vi "Test_API_AsynchShutdown_NoErrorEventsCaptured.vi"(8 "error in (no error)":errorcluster, 11 "TestCase in":refnum<class "TestLocalLogInstance.lvclass">) -> (0 "error out":errorcluster, 3 "TestCase out":refnum<class "TestLocalLogInstance.lvclass">)   [LabVIEW 2019, in "TestLocalLogInstance.lvclass"]
uses:
  TestLocalLogInstance.lvclass
  Source/Composed Log/Types/Log Level.ctl
  Source/LVQueue Sink/LVQueue Sink.lvclass/LVQueue Sink.ctl
  Source/Composed Log/LoggerReference/LoggerReference.lvclass/LoggerReference.ctl
  e881e85d-d289-450a-a3bf-8e76de4143bc.vi
  145e8f28-aa7d-4165-8971-95667389dd01.vi
  Source/Composed Log/LoggerReference/Return Aggregate Queues.vi
  Source/Composed Log/LoggerReference/Add Aggregate Log.vi
  e881e85d-d289-450a-a3bf-8e76de4143bc.vi/56849bd9-e0f3-42e2-9e62-1194216846a3.vi
  Source/Composed Log/LoggerReference/Log.vi
  Source/Composed Log/LoggerReference/Get Valid Event Time.vi
  Source/Composed Log/LoggerReference/Send Add Sink.vi
  Source/Composed Log/LoggerReference/Remove Stale Logs.vi
  Source/LVQueue Sink/LVQueue Sink.lvclass
  C:/CS/Log/Source/Composed Log/Log Sink/Log Sink.lvclass
  Source/Composed Log/Application Logger/Launch Worker Loop.vi
  Source/Composed Log/LoggerReference/Initialize Logger Instance.vi
  Source/Composed Log/LoggerReference/LoggerReference.lvclass
  Source/Composed Log/IErrorFormat/IErrorFormat.lvclass
  Source/Composed Log/Log Sink/Log Sink.lvclass
  <vilib>/addons/_JKI Toolkits/VI Tester/TestCase.llb/TestCase.lvclass
  Source/Composed Log/Composed Log.lvlib
  C:/Program Files (x86)/National Instruments/LabVIEW 2019/vi.lib/addons/_JKI Toolkits/VI Tester/TestCase.llb/TestCase.lvclass
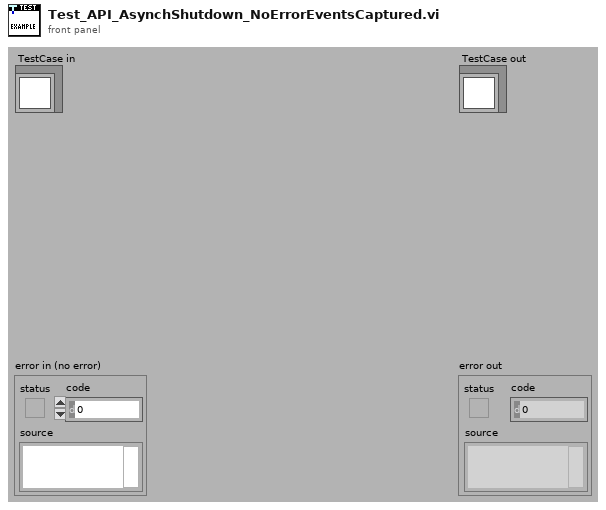
[diagram p1: front panel]
types:
  T1 = typedef "Composed Log.lvlib/Log Level.ctl" = enum16{"Debug", "Info", "Warning", "Error", "Critical"}
  T2 = typedef "Composed Log.lvlib/Log Packet.ctl" = cluster{"Data To Log":string, "Source":string, "Event Level":T1, "Event Time":timestamp}
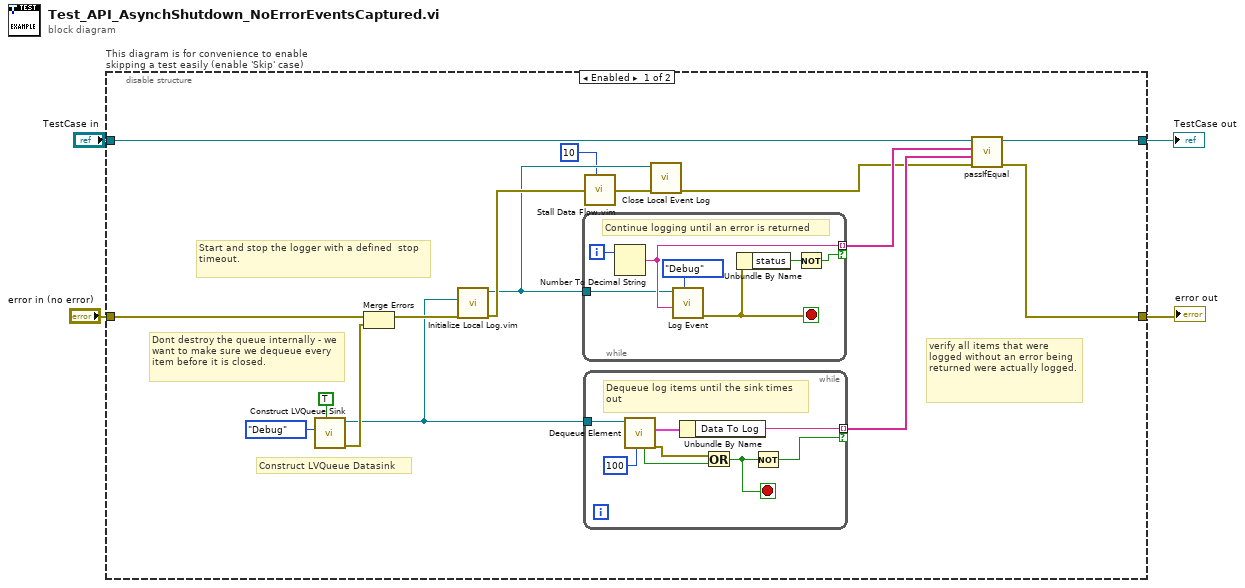
[diagram p0: block diagram]
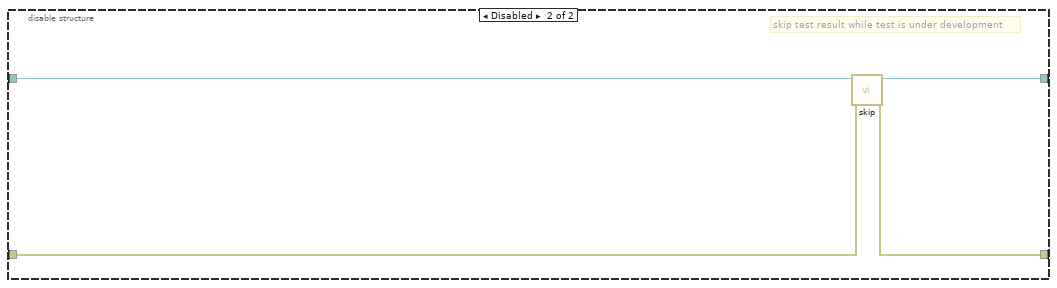
[diagram p2: hidden frame]
diagram:
  n1 = disable-structure "This diagram is for convenience to enable skipping a test easily (enable 'Skip' case)" shown="Enabled" {
    disable-tunnel: "TestCase in" -> [w18 w39]
    disable-tunnel: [w19 w37] -> w1
    disable-tunnel: [w17 w38] -> w3
    disable-tunnel: "error in (no error)" -> [w20 w36]
    frame Enabled {
      # "Dont destroy the queue internally - we want to make sure we dequeue every item before it is closed."
      # "verify all items that were logged without an error being returned were actually logged."
      # "Construct LVQueue Datasink"
      # "Start and stop the logger with a defined  stop timeout."
      n2 = call "Construct LVQueue Sink.vi"("User Shutdown? (F)"=TRUE, "LogLevel"=Log_Level."Debug") -> ("error out"=w15:errorcluster, "LVQueue Sink out"=w10:refnum<class "LVQueue Sink.lvclass">)  [unwired: 8 in]
      n3 = Merge Errors(w20, w15) -> (w11:errorcluster)
      n4 = call "Initialize Local Log.vim"("error in (no error)"=w11, "Startup Sink(s)"=w10) -> ("error out"=w9:errorcluster, "Log Instance Reference"=w8:refnum<class "LoggerReference.lvclass">)  [unwired: 7 in, 1 out]
      n5 = while {
        tunnel: [w30] -> w14 mode=indexing if=w31
        tunnel: w8 -> [w29]
        i -> [w34]
        stop <- w33 stop-if-true
        # "Continue logging until an error is returned"
        n6 = Number To Decimal String(number=w34) -> (decimal integer string=w30:string)  [unwired: 1 in]
        n7 = call "Log Event.vi"("Event Level"=Log_Level."Debug", "Data To Log"=w30, "Log Instance"=w29) -> ("error out"=w33:errorcluster)  [unwired: 7 in, 1 out]
        n8 = Unbundle By Name(w33) -> ("status"=w32:bool)
        n9 = Not(x=w32) -> (.not. x?=w31:bool)
      }
      n10 = while {
        tunnel: w10 -> [w28]
        tunnel: [w25] -> w12 mode=indexing if=w22
        stop <- w21 stop-if-true
        # "Dequeue log items until the sink times out"
        n11 = call "Dequeue Element.vi"("timeout in ms (-1)"=100, "LVQueue Sink in"=w28) -> ("error out"=w23:errorcluster, "Log Packet"=w26:T2, "Timed Out?"=w24:bool)  [unwired: 6 in, 1 out]
        n12 = Unbundle By Name(w26) -> ("Data To Log"=w25:string)
        n13 = Or(x=w23, y=w24) -> (x .or. y?=w21:bool)
        n14 = Not(x=w21) -> (.not. x?=w22:bool)
      }
      n15 = call "Stall Data Flow.vim"("value in"=w9, "milliseconds to wait"=u32 10) -> ("value out"=w6:errorcluster)  [unwired: 1 out]
      n16 = call "Close Local Event Log.vi"("error in (no error)"=w6, "Log Instance"=w8) -> ("error out"=w7:errorcluster)  [unwired: 9 in]
      n17 = call-dynamic "passIfEqual.vi"("error in (no error)"=w7, "y"=w12, "x"=w14, "TestCase in"=w18) -> ("error out"=w17:errorcluster, "TestCase out"=w19:refnum<class "TestLocalLogInstance.lvclass">)  [unwired: 6 in]
    }
    frame Disabled {
      # "skip test result while test is under development"
      n18 = call <vilib>:"skip.vi"("error in (no error)"=w36, "TestCase in"=w39) -> ("error out"=w38:errorcluster, "TestCase out"=w37:refnum<class "TestLocalLogInstance.lvclass">)  [unwired: 8 in]
    }
  }
  "error out" <- w3
  "TestCase out" <- w1
